vi "AllenBradlenLightSensor-DigitalInput.vi"() -> ()   [LabVIEW 2020]
doc: "This example shows how to use a digital line to read a limit switch."
uses:
  <vilib>/Rock Robotics/SystemInterfaces/DIO/FPGA_DIOChannel.ctl
  <vilib>/Rock Robotics/WPI/Switch/WPI_SwitchOpenLimit.vi
panel:
  out "Switch Value":bool
  in  "DIO Channel":T1=enum."DIO 8"
  in  "stop":bool
  in  "Normally Closed":bool=TRUE
  # "Set these inputs before running."
  # "roboRIO Wiring Diagram"
  # "Limit\nSwitch"
  # "COM"
  # "NC"
  # "NO"
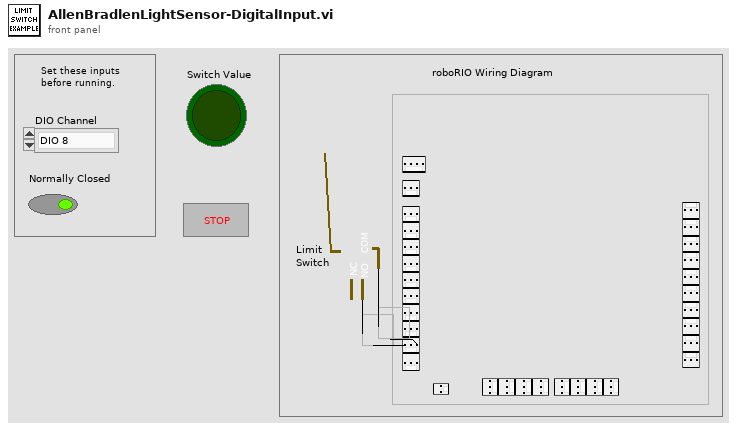
[diagram p1: front panel]
types:
  T1 = typedef "FPGA_DIOChannel.ctl" = enum8{"DIO 0", "DIO 1", "DIO 2", "DIO 3", "DIO 4", "DIO 5", "DIO 6", "DIO 7", "DIO 8", "DIO 9", "DIO MXP 0", "DIO MXP 1", "DIO MXP 2", "DIO MXP 3", "DIO MXP 4", "DIO MXP 5", "DIO MXP 6", "DIO MXP 7", "DIO MXP 8", "DIO MXP 9", "DIO MXP 10", "DIO MXP 11", "DIO MXP 12", "DIO MXP 13", "DIO MXP 14", "DIO MXP 15", "SPI Port CS1", "SPI Port CS2", "SPI Port CS3", "SPI Port MISO", "SPI Port MOSI", "Invalid"}
  T2 = typedef "WPI_SwitchDevRef.ctl" = cluster{"DevStatus":errorcluster, "DIO Channel":T1, "CntIndex":T3, "Normally Closed":bool}
  T3 = typedef "FPGA_CounterCtrSystemIndex.ctl" = enum8{"Ctr 0", "Ctr 1", "Ctr 2", "Ctr 3", "Ctr 4", "Ctr 5", "Ctr 6", "Ctr 7", "Invalid"}
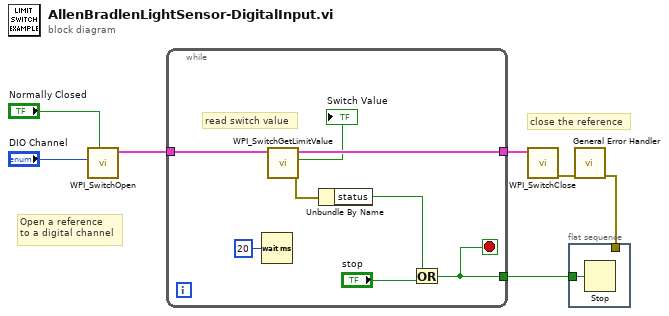
[diagram p0: block diagram]
diagram:
  # "Open a reference\nto a digital channel"
  # "close the reference"
  n1 = call-poly <vilib>:"WPI_SwitchOpen.vi"("Normally Closed"="Normally Closed", "DIO Channel"="DIO Channel") -> ("SwitchDevRef"=w3:T2)  [unwired: 8 in, 1 out]
  n2 = while {
    tunnel: [w15] -> w7
    tunnel: w3 -> [w9]
    tunnel: [w8] -> w2
    stop <- w8 stop-if-true
    # "read switch value"
    n3 = Wait (ms)(milliseconds to wait=u32 20) -> ()  [unwired: 1 out]
    n4 = call <vilib>:"WPI_SwitchGetLimitValue.vi"("SwitchDevRef"=w9) -> ("error out"=w14:errorcluster, "Switch Pressed"=→"Switch Value":bool, "SwitchDevRef"=w15:T2)  [unwired: 8 in]
    n5 = Unbundle By Name(w14) -> ("status"=w13:bool)
    n6 = Or(x=w13, y="stop") -> (x .or. y?=w8:bool)
  }
  n7 = call <vilib>:"WPI_SwitchClose.vi"("SwitchDevRef"=w7) -> ("error out"=w6:errorcluster)  [unwired: 10 in]
  n8 = flat-sequence {
    tunnel: w2 -> [w16]
    tunnel: w1 -> [_]
    frame #0 {
      n9 = Stop(stop? (T)=w16) -> ()
    }
  }
  n10 = call <vilib>:"General Error Handler.vi"("error in (no error)"=w6) -> ("error out"=w1:errorcluster)  [unwired: 10 in, 4 out]
